vi "CompareDevices_queued.vi"(9 "New Dev queue":refnum<queue>, 10 "Old Dev queue":refnum<queue>) -> (2 "compatible?":bool, 4 "New Dev queue invalid?":bool, 5 "Old Dev queue invalid?":bool)   [LabVIEW 2013]
doc: "This utility checks if two device arrays are \"compatible.\" \n\nCompatible arrays have the same number of devices, each of which matches in device class and column classes. No private data (such as table SWI, column \"functionality\", etc.) is checked.\n\nThe comparison is done linearly through the arrays by device and is stopped upon finding the first incompatibility. If a size mismatch is encountered, the internal monitors \"<array> index\" are set to -1. Otherwise, they record the index where a class mismatch occured; if no mismatch is found, index then contains the length of each matched column array."
uses:
  Device/Device.lvclass
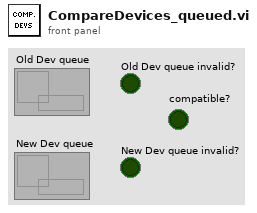
[diagram p1: front panel]
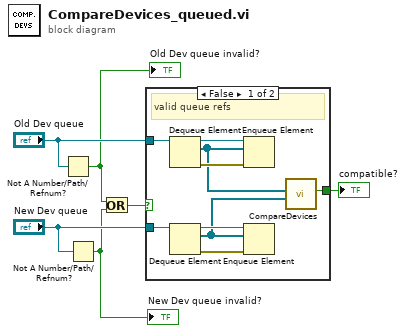
[diagram p0: block diagram]
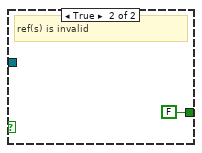
[diagram p2: hidden frame]
diagram:
  n1 = Not A Number/Path/Refnum?(number/path/refnum="Old Dev queue") -> (NaN/Path/Refnum?=w2:bool)
  "Old Dev queue invalid?" <- w2
  n2 = Not A Number/Path/Refnum?(number/path/refnum="New Dev queue") -> (NaN/Path/Refnum?=w3:bool)
  "New Dev queue invalid?" <- w3
  n3 = Or(x=w2, y=w3) -> (x .or. y?=w1:bool)
  n4 = case shown="False" w1 {
    tunnel: [w9 FALSE ("compatible?")] -> w6
    tunnel: "Old Dev queue" -> [w8 _]
    tunnel: "New Dev queue" -> [w7 _]
    frame False {
      # "valid queue refs"
      n5 = Dequeue Element(queue=w8) -> (queue out=w15:refnum<queue>, element=w11:refnum<class "Device.lvclass">[], error out=w14:errorcluster)  [unwired: 2 in, 1 out]
      n6 = Dequeue Element(queue=w7) -> (queue out=w12:refnum<queue>, element=w10:refnum<class "Device.lvclass">[], error out=w13:errorcluster)  [unwired: 2 in, 1 out]
      n7 = Enqueue Element(queue=w15, element=w11, error in (no error)=w14) -> ()  [unwired: 1 in, 3 out]
      n8 = Enqueue Element(queue=w12, element=w10, error in (no error)=w13) -> ()  [unwired: 1 in, 3 out]
      n9 = call "CompareDevices.vi"("New Dev array"=w10, "Old Dev array"=w11) -> ("compatible?"=w9:bool)  [unwired: 9 in]
    }
    frame True {
      # "ref(s) is invalid"
    }
  }
  "compatible?" <- w6
